vi "Get DDG Lite Inter Pulse Delay.vi"(10 "fDelay":sgl, 11 "channel":u32(ring)=65535 items=["AT_DDGLite_ChannelA"=1073741824, "AT_DDGLite_ChannelB"=1073741825, "AT_DDGLite_ChannelC"=1073741826]) -> (2 "fDelay out":sgl, 3 "function return":u32)   [LabVIEW 2018, in "AndorSDK.lvlib"]
doc: "EXPNETTYPE unsigned int WINAPI GetDDGLiteInterPulseDelay(AT_DDGLiteChannelId channel, float * fDelay);"
uses:
  AndorSDK.lvlib
  ATMCD32D.dll
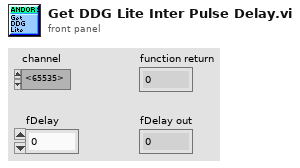
[diagram p1: front panel]
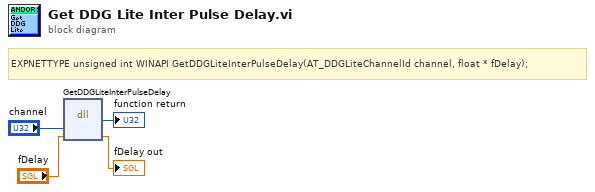
[diagram p0: block diagram]
diagram:
  # "EXPNETTYPE unsigned int WINAPI GetDDGLiteInterPulseDelay(AT_DDGLiteChannelId channel, float * fDelay);"
  n1 = dll-call lib="PTH2babs E\nPersönliches02 - Arbeit03-HiwijobsLabviewCodelibANDOR\tAndor SDK\nATMCD32D.*" fn="GetDDGLiteInterPulseDelay"("channel"="channel", "fDelay"="fDelay") -> (→"function return":u32, "fDelay"=→"fDelay out":sgl)  [unwired: 4 in, 2 out]
